vi "Host4.vi"() -> ()   [LabVIEW 2025]
uses:
  <vilib>/numeric/Random Number (Range) U64.vi
  <vilib>/Analysis/baseanly.llb/Real Dot Product.vi
  <vilib>/Analysis/baseanly.llb/Real A x B.vi
  <vilib>/numeric/sub_Random U32.vi
  <vilib>/Analysis/Matrix/Numeric/Conversions/Matrix To Array - RM.vi
  <vilib>/FPGAPlugInAG/cRIO-9033/niLvFpga_Open_cRIO-9033.vi
  <vilib>/rvi/interface/common/dynamic/niFpgaDynamicAddResources.vi
  <vilib>/FPGAPlugInAG/Dynamic/niLvFpga_Run_Dynamic.vi
  <vilib>/Utility/error.llb/Error Cluster From Error Code.vi
  <vilib>/rvi/errors/niLvFpgaAdjustHostInterfaceError.vi
  <vilib>/FPGAPlugInAG/Dynamic/niLvFpga_Close_Dynamic.vi
  <vilib>/rvi/interface/nirviOpenFPGA/nirviOpenFPGA.xnode
  FPGA Bitfiles/dotplot9033_FPGATarget_Target4_KK3y63-7e1g.lvbitx
  Target4.vi
  <vilib>/rvi/interface/nirviMethod/nirviMethod.xnode
  <vilib>/rvi/interface/nirviCloseFPGA/nirviCloseFPGA.xnode
  <vilib>/rvi/errors/niLvFpgaMergeErrorWithErrorCode.vi
  <vilib>/FPGAPlugInAG/Dynamic/niLvFpga_ReadFifo_Dynamic.vi
  <vilib>/Analysis/NI_AALBase.lvlib
  <vilib>/Analysis/Matrix/NI_Matrix.lvlib
panel:
  out "FIFO C Output":fxp<+/-,32,16>[](array[numeric])
  out "FIFO A Input":fxp<+/-,32,16>[](array[numeric])
  out "FIFO B Input":fxp<+/-,32,16>[](array[numeric])
  out "X * Y":fxp<+/-,64,32>
  out "elements in B":i32
  out "elements in A":i32
  out "sum of error":dbl
  out "C - FPGA code":fxp<+/-,32,16>[][](array[numeric])
  out "elements in C":i32
  out "C - Real":dbl[][](array[numeric])
  out "B":fxp<+/-,32,16>[][](array[numeric])
  out "A":fxp<+/-,32,16>[][](array[numeric])
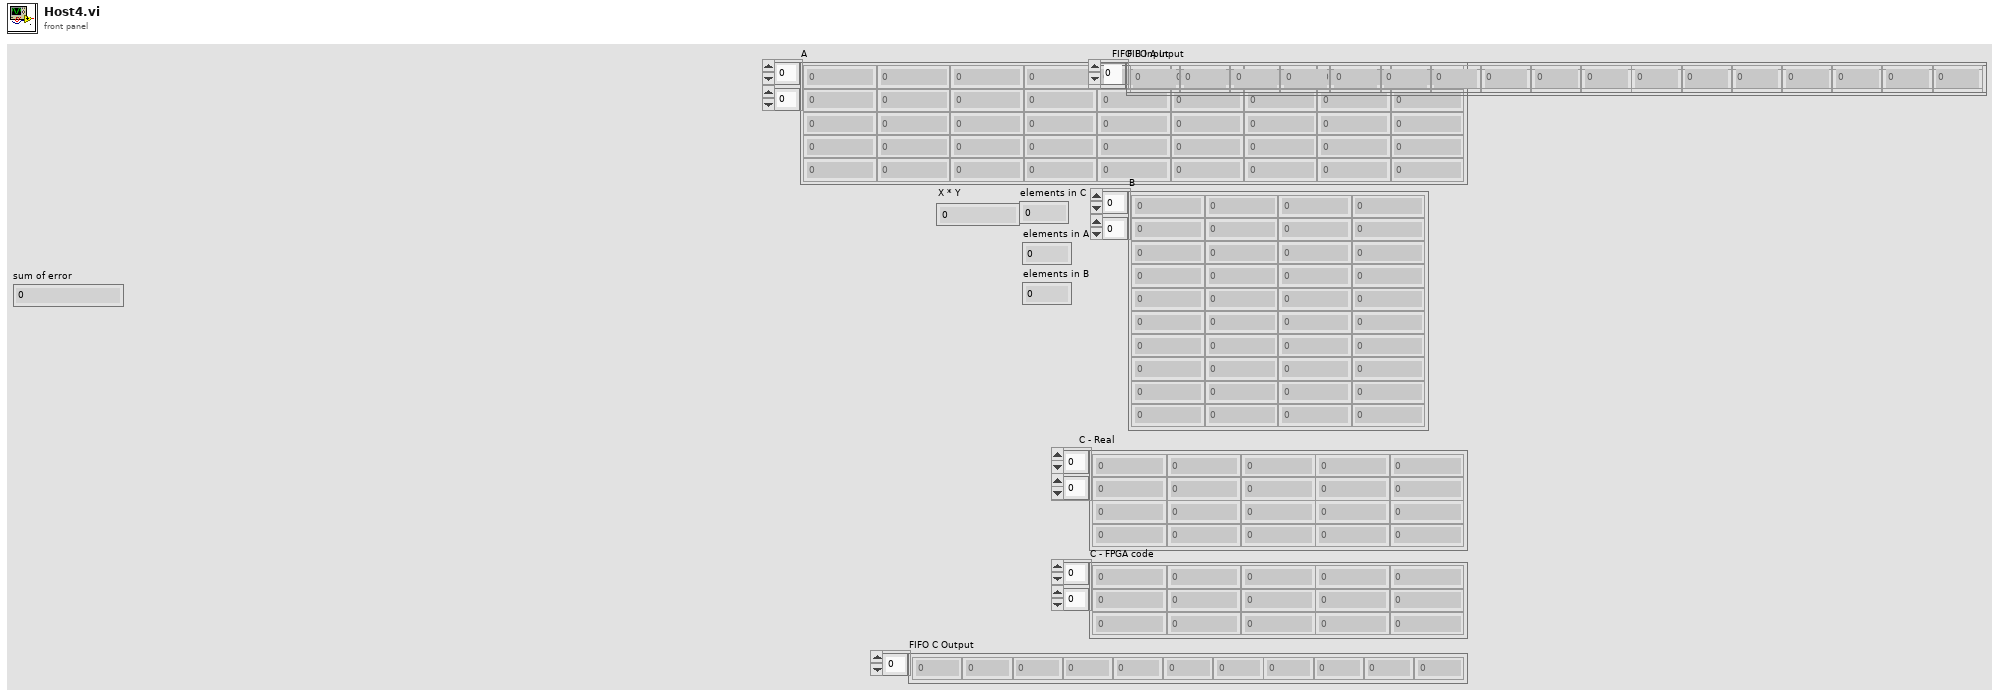
[diagram p1: front panel]
types:
  T1 = typedef "NI_Matrix.lvlib/RealMatrix.ctl" = dbl[][]
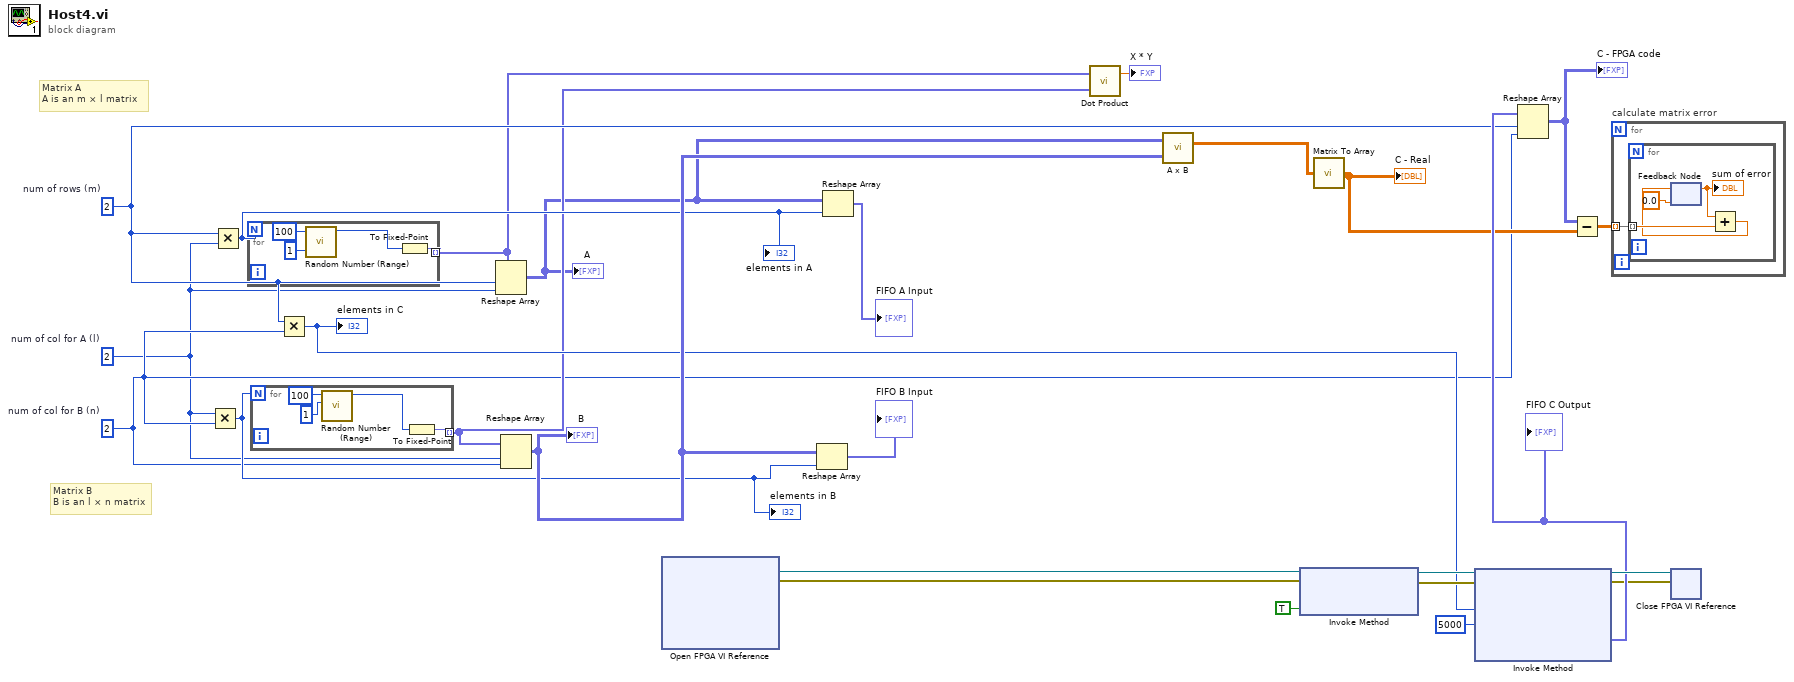
[diagram p0: block diagram]
diagram:
  w6 = 2  # num of col for B (n)
  w5 = 2  # num of col for A (l)
  w15 = 2  # num of rows (m)
  # "Matrix B\nB is an l × n matrix"
  # "Matrix A\nA is an m × l matrix"
  n1 = Multiply(x=w5, y=w6) -> (x*y=w12:i32)
  "elements in B" <- w12
  n2 = Multiply(x=w15, y=w5) -> (x*y=w20:i32)
  "elements in A" <- w20
  n3 = for {
    N: w20 -> [_]
    tunnel: [w30] -> w11 mode=indexing
    n4 = call-poly <vilib>:"Random Number (Range).vi"("lower bound (0)"=u64 1, "upper bound (100)"=u64 100) -> ("number"=w29:u64)  [unwired: 9 in]
    n5 = To Fixed-Point(number=w29) -> (fixed-point=w30:fxp<+,64,64>)  [unwired: 1 in]
  }
  n6 = for {
    N: w12 -> [_]
    tunnel: [w34] -> w10 mode=indexing
    n7 = call-poly <vilib>:"Random Number (Range).vi"("lower bound (0)"=u64 1, "upper bound (100)"=u64 100) -> ("number"=w31:u64)  [unwired: 9 in]
    n8 = To Fixed-Point(number=w31) -> (fixed-point=w34:fxp<+,64,64>)  [unwired: 1 in]
  }
  n9 = Multiply(x=w15, y=w6) -> (x*y=w13:i32)
  "elements in C" <- w13
  n10 = Reshape Array(w11, w15, w5) -> (w7:fxp<+,64,64>[][])
  "A" <- w7
  n11 = Reshape Array(w10, w5, w6) -> (w22:fxp<+,64,64>[][])
  "B" <- w22
  n12 = xnode "Open FPGA VI Reference"() -> ("FPGA VI Reference Out"=w2:refnum<k20>, "error out"=w1:errorcluster)  [unwired: 2 in]
  n13 = Reshape Array(w22, w12) -> (→"FIFO B Input":fxp<+,64,64>[])
  n14 = Reshape Array(w7, w20) -> (→"FIFO A Input":fxp<+,64,64>[])
  n15 = call-poly <vilib>:"Dot Product.vi"("Y Vector"=w10, "X Vector"=w11) -> ("X * Y"=→"X * Y":dbl)  [unwired: 1 out]
  n16 = call-poly <vilib>:"A x B.vi"("B"=w22, "A"=w7) -> ("A x B"=w21:T1)  [unwired: 1 out]
  n17 = xnode "Invoke Method"("FPGA VI Reference In"=w2, "error in"=w1, "Wait Until Done (F)"=TRUE) -> ("FPGA VI Reference Out"=w25:refnum<k20>, "error out"=w24:errorcluster)
  n18 = call-poly <vilib>:"Matrix To Array.vi"("Real Matrix"=w21) -> ("Real 2D Array"=w14:dbl[][])
  "C - Real" <- w14
  n19 = xnode "Invoke Method"("FPGA VI Reference In"=w25, "error in"=w24, "Number of Elements"=w13, "Timeout (ms)"=5000) -> ("FPGA VI Reference Out"=w23:refnum<k20>, "error out"=w8:errorcluster, "Data"=w16:fxp<+/-,32,16>[])  [unwired: 1 out]
  "FIFO C Output" <- w16
  n20 = Reshape Array(w16, w15, w6) -> (w18:fxp<+/-,32,16>[][])
  "C - FPGA code" <- w18
  n21 = Subtract(x=w18, y=w14) -> (x-y=w17:dbl[][])
  n22 = for "calculate matrix error" {
    tunnel: w17 -> [w35] mode=indexing
    n23 = for {
      tunnel: w35 -> [w39] mode=indexing
      n24 = feedback #1(0.0) -> (w37:dbl)
      "sum of error" <- w37
      n25 = Add(x=w37, y=w39) -> (x+y=w38:dbl)
      n26 = feedback-in #1(w38) -> ()
    }
  }
  n27 = xnode "Close FPGA VI Reference"("FPGA VI Reference In"=w23, "error in"=w8) -> ()  [unwired: 1 out]
